vi "test_myRIO_Exp_tLoop.vi"(7 "input_error":errorcluster, 9 "input_Threshold":bool, 10 "input_timestamp":timestamp, 11 "input_state":T1=enum."setSettings_Laser") -> (1 "output_Threshold":bool, 2 "output_duration":dbl, 5 "error out":errorcluster)   [LabVIEW 2014]
uses:
  myRIO_BRig_RT__Case_Exp_stateList.ctl
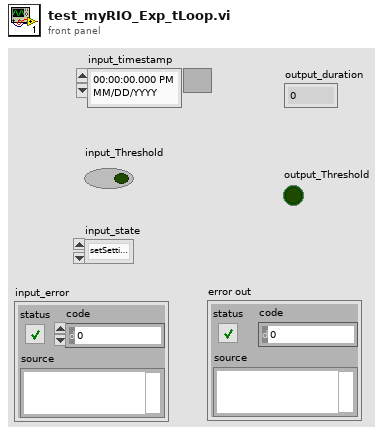
[diagram p1: front panel]
types:
  T1 = typedef "myRIO_BRig_RT__Case_Exp_stateList.ctl" = enum16{"Start1", "Start2", "Start3", "saveSettings1", "saveSettings2", "saveSettings3", "saveSettings4", "saveSettings_LC_ENL_l1", "saveSettings_LC_ENL_l2", "saveSettings_LC_Cue_l1", "saveSettings_LC_Cue_l2", "saveSettings6_LC_l1_Other", "SaveSettings6_LC_l2_Other", "setSettings_Audio", "setSettings_Laser", "initBlock_pre", "initBlock", "initBlock2", "initBlock_post", "initTrial_pre", "initTrial", "initTrial2", "initTrial3", "initTrial4", "initTrial_LC_ENL1", "initTrial_LC_Cue1", "initTrial_LC_Cue1_2", "initTrial_LC_Sel", "initTrial_post", "ENL1_pre", "ENL1", "ENL1_post", "ENL1Penalty_pre", "ENL1Penalty", "ENL2_pre", "ENL2", "ENL2Penalty_pre", "ENL2Penalty", "Cue1_pre", "Cue1", "Cue1_post", "Cue1Penalty_pre", "Cue1Penalty", "Cue2_pre", "Cue2", "Cue2Penalty_pre", "Cue2Penalty", "Selection_pre", "Selection", "Select_post", "SelectReward_pre", "SelectReward", "SelectRewardPost_pre", "SelectRewardPost", "SelectWrong_pre", "SelectWrong", "SelectWrong_post", "SelectTimeout_pre", "SelectTimeout", "SelectTimeout_post", "endTrial_pre", "endTrial1", "endTrial2", "endTrial3", "endTrial_post", "endBlock_pre", "endBlock", "endBlock_post", "endExp", "commConnect", "commUpload_pre", "commUpload_dataBlock", "commUpload_dataCurrent", "commUpload_dataExp", "commUpload_dataLC", "commUpload_dataTrial", "commUpload_post", "saveData_pre", "saveData_dataBlock", "saveData_dataCurrent", "saveData_dataExp", "saveData_dataLC", "saveData_dataTrial", "saveData_post", "empty_endBlock1", "empty_endBlock2", "empty_endTrial1", "empty_endTrial2", "empty_endTrial3", "empty_endTrial4", "empty_endTrial5", "dummyState", "dummyState_endBlock"}
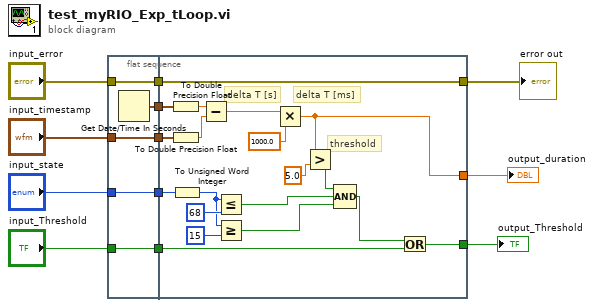
[diagram p0: block diagram]
diagram:
  n1 = flat-sequence {
    tunnel: "input_error" -> [w17]
    tunnel: "input_timestamp" -> [w15]
    tunnel: [w17] -> w12
    tunnel: [w16] -> w11
    tunnel: [w15] -> w10
    tunnel: "input_Threshold" -> [w14]
    tunnel: [w14] -> w9
    tunnel: [w13] -> w2
    tunnel: "input_state" -> [w13]
    tunnel: [w36] -> w7
    tunnel: w12 -> [w36]
    tunnel: w11 -> [w35]
    tunnel: w10 -> [w33]
    tunnel: w9 -> [w28]
    tunnel: [w27] -> w5
    tunnel: [w26] -> w4
    tunnel: w2 -> [w25]
    frame #0 {
      n2 = Get Date/Time In Seconds() -> (seconds since 1Jan1904=w16:timestamp)
    }
    frame #1 {
      # "threshold"
      # "delta T [ms]"
      # "delta T [s]"
      n3 = To Double Precision Float(number=w35) -> (double precision float=w34:dbl)
      n4 = To Double Precision Float(number=w33) -> (double precision float=w32:dbl)
      n5 = To Unsigned Word Integer(number=w25) -> (unsigned 16bit integer=w20:u16)
      n6 = Subtract(x=w34, y=w32) -> (x-y=w31:dbl)
      n7 = Less Or Equal?(x=w20, y=u16 68) -> (x <= y?=w23:bool)
      n8 = Greater Or Equal?(x=w20, y=u16 15) -> (x >= y?=w18:bool)
      n9 = Multiply(x=w31, y=1000.0) -> (x*y=w26:dbl)
      n10 = Greater?(x=w26, y=5.0) -> (0:w24:bool)
      n11 = Compound Arithmetic op=AND(w24, w23, w18) -> (w22:bool)
      n12 = Or(x=w22, y=w28) -> (x .or. y?=w27:bool)
    }
  }
  "error out" <- w7
  "output_Threshold" <- w5
  "output_duration" <- w4
